vi "flow meter test.vi"() -> ()   [LabVIEW 2013]
uses:
  <vilib>/Platform/TimedLoop/XDataNode/timing_clust.ctl
  <vilib>/Platform/TimedLoop/XDataNode/nitl_modes.ctl
  <vilib>/Platform/TimedLoop/XDataNode/wakeup.ctl
  <vilib>/rvi/Emulation/niFpgaSctlEmulationGetInTimedLoop.vi
  <vilib>/rvi/Emulation/niFpgaEmulationReportErrorSimple.vi
  <vilib>/rvi/Emulation/niFpgaGetClockAttributes.vi
  <vilib>/rvi/Emulation/niFpgaCriticalErrorInLSC.vi
  <vilib>/rvi/eio/common/nirviEmuTemplateMethod_errors.vi
  <vilib>/Platform/TimedLoop/XDataNode/XDataNode.xnode
  <vilib>/eio/EIONode/EIONode.xnode
  <vilib>/Platform/TimedLoop/XDataNode/XDNodeRunTimeDep.lvlib
panel:
  out "Period 6 (ticks)":u32
  out "Period 5 (ticks)":u32
  out "Period 4 (ticks)":u32
  out "Period 3 (ticks)":u32
  out "Period 2 (ticks)":u32
  in  "Max Period (ticks)":u32
  out "Period 1 (ticks)":u32
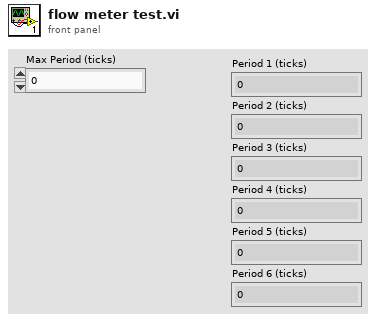
[diagram p1: front panel]
types:
  T1 = typedef "XDNodeRunTimeDep.lvlib/timing_clust.ctl" = cluster{"Expected End [f-1]":u64, "Actual End [f-1]":u64, "Finished Late? [f-1]":bool, "Expected End [i-1]":u64, "Actual End [i-1]":u64, "Finished Late? [i-1]":bool, "Expected Start [i]":u64, "Actual Start [i]":u64, "Expected Start [f]":u64, "Actual Start [f]":u64, "Source Name":string, "Structure Name":string, "Period":i64, "Deadline":i64, "Offset":i64, "Start":i64, "Priority":i32, "Timeout":i32, "Mode":T2, "Wakeup Reason":T3, "Error":errorcluster, "Source Type":string, "Secondary Source Type":string, "Global End Time":u64, "Global Start Time":u64, "Frame Duration":u64, "Iteration Duration":u64, "Assigned CPU":i32, "I/O Scan Engine Mode":u32}
  T2 = typedef "XDNodeRunTimeDep.lvlib/nitl_modes.ctl" = enum32{"No Change", "Process missed periods, maintain original phase", "Discard missed periods, maintain original phase", "Process missed periods, ignore original phase", "Discard missed periods, ignore original phase"}
  T3 = typedef "XDNodeRunTimeDep.lvlib/wakeup.ctl" = enum32{"Normal", "Aborted", "Asynchronous wakeup", "Timing source error", "Timed loop error", "Timeout"}
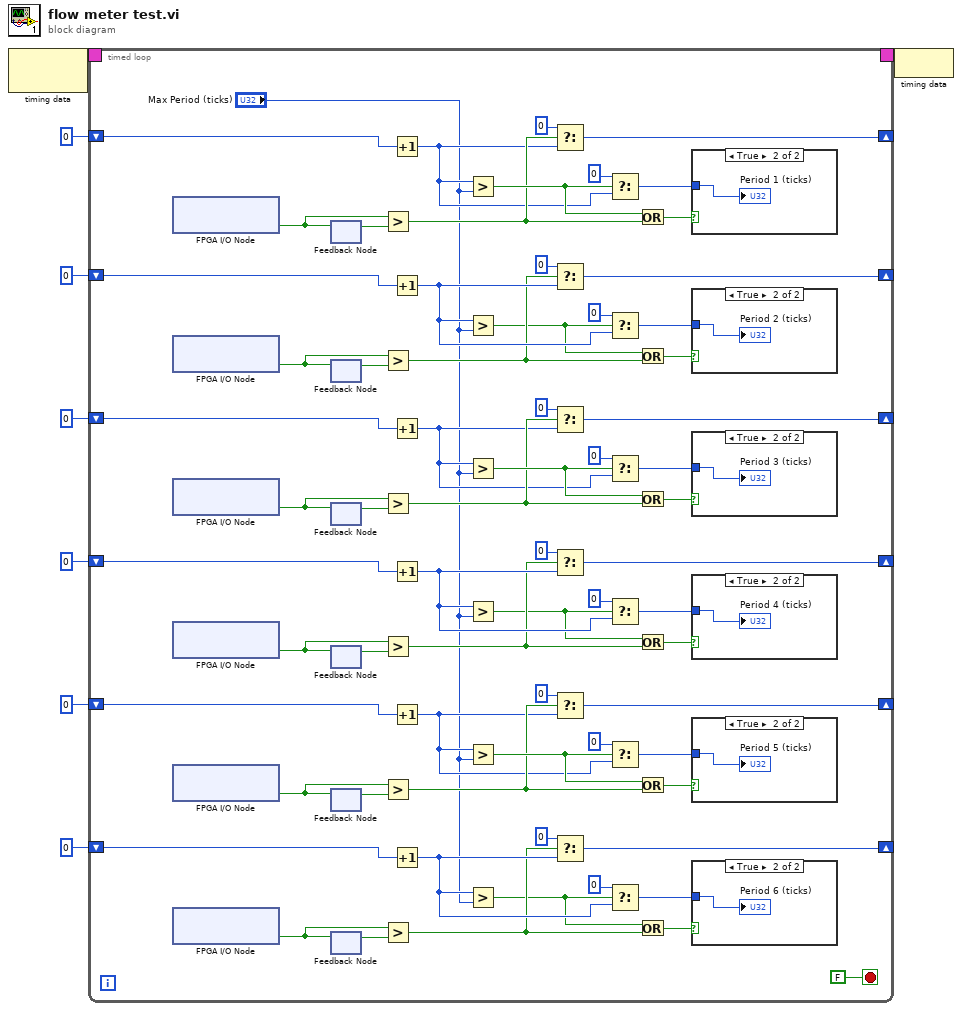
[diagram p0: block diagram]
diagram:
  n1 = node-c288() -> (w8:T1)  [unwired: 1 in]
  n2 = timed-loop {
    timing: w8 -> [_]
    timing-out: [_] -> w7
    shift-right: [w67] -> _
    shift-left: u32 0 ("f") -> [w66]
    shift-right: [w62] -> _
    shift-left: u32 0 ("f") -> [w63]
    shift-right: [w45] -> _
    shift-left: u32 0 ("f") -> [w44]
    shift-right: [w40] -> _
    shift-left: u32 0 ("f") -> [w41]
    shift-right: [w23] -> _
    shift-left: u32 0 ("f") -> [w22]
    shift-right: [w18] -> _
    shift-left: u32 0 ("f") -> [w19]
    stop <- FALSE stop-if-true
    n3 = xnode "FPGA I/O Node"() -> ("RMC/DIO32"=w75:bool)  [unwired: 1 in, 1 out]
    n4 = xnode "FPGA I/O Node"() -> ("RMC/DIO33"=w54:bool)  [unwired: 1 in, 1 out]
    n5 = xnode "FPGA I/O Node"() -> ("RMC/DIO34"=w53:bool)  [unwired: 1 in, 1 out]
    n6 = xnode "FPGA I/O Node"() -> ("RMC/DIO35"=w32:bool)  [unwired: 1 in, 1 out]
    n7 = xnode "FPGA I/O Node"() -> ("RMC/DIO36"=w31:bool)  [unwired: 1 in, 1 out]
    n8 = xnode "FPGA I/O Node"() -> ("RMC/DIO37"=w10:bool)  [unwired: 1 in, 1 out]
    n9 = feedback-in #1(w75) -> ()
    n10 = feedback #1() -> (w74:bool)  [unwired: 1 in]
    n11 = feedback #2() -> (w55:bool)  [unwired: 1 in]
    n12 = feedback-in #2(w54) -> ()
    n13 = feedback #3() -> (w52:bool)  [unwired: 1 in]
    n14 = feedback-in #3(w53) -> ()
    n15 = feedback #4() -> (w33:bool)  [unwired: 1 in]
    n16 = feedback-in #4(w32) -> ()
    n17 = feedback #5() -> (w30:bool)  [unwired: 1 in]
    n18 = feedback-in #5(w31) -> ()
    n19 = feedback #6() -> (w11:bool)  [unwired: 1 in]
    n20 = feedback-in #6(w10) -> ()
    n21 = Greater?(x=w75, y=w74) -> (0:w69:bool)
    n22 = Greater?(x=w54, y=w55) -> (0:w60:bool)
    n23 = Greater?(x=w53, y=w52) -> (0:w47:bool)
    n24 = Greater?(x=w32, y=w33) -> (0:w38:bool)
    n25 = Greater?(x=w31, y=w30) -> (0:w25:bool)
    n26 = Greater?(x=w10, y=w11) -> (0:w16:bool)
    n27 = Increment(x=w66) -> (x+1=w65:u32)
    n28 = Increment(x=w63) -> (x+1=w64:u32)
    n29 = Increment(x=w44) -> (x+1=w43:u32)
    n30 = Increment(x=w41) -> (x+1=w42:u32)
    n31 = Increment(x=w22) -> (x+1=w21:u32)
    n32 = Increment(x=w19) -> (x+1=w20:u32)
    n33 = Greater?(x=w65, y="Max Period (ticks)") -> (0:w71:bool)
    n34 = Greater?(x=w64, y="Max Period (ticks)") -> (0:w58:bool)
    n35 = Greater?(x=w43, y="Max Period (ticks)") -> (0:w49:bool)
    n36 = Greater?(x=w42, y="Max Period (ticks)") -> (0:w36:bool)
    n37 = Greater?(x=w21, y="Max Period (ticks)") -> (0:w27:bool)
    n38 = Greater?(x=w20, y="Max Period (ticks)") -> (0:w14:bool)
    n39 = Select(t=u32 0 ("f"), s=w69, f=w65) -> (s? t:f=w67:u32)
    n40 = Select(t=u32 0 ("f"), s=w60, f=w64) -> (s? t:f=w62:u32)
    n41 = Select(t=u32 0 ("f"), s=w47, f=w43) -> (s? t:f=w45:u32)
    n42 = Select(t=u32 0 ("f"), s=w38, f=w42) -> (s? t:f=w40:u32)
    n43 = Select(t=u32 0 ("f"), s=w25, f=w21) -> (s? t:f=w23:u32)
    n44 = Select(t=u32 0 ("f"), s=w16, f=w20) -> (s? t:f=w18:u32)
    n45 = Select(t=u32 0 ("f"), s=w71, f=w65) -> (s? t:f=w73:u32)
    n46 = Select(t=u32 0 ("f"), s=w58, f=w64) -> (s? t:f=w56:u32)
    n47 = Select(t=u32 0 ("f"), s=w49, f=w43) -> (s? t:f=w51:u32)
    n48 = Select(t=u32 0 ("f"), s=w36, f=w42) -> (s? t:f=w34:u32)
    n49 = Select(t=u32 0 ("f"), s=w27, f=w21) -> (s? t:f=w29:u32)
    n50 = Select(t=u32 0 ("f"), s=w14, f=w20) -> (s? t:f=w12:u32)
    n51 = Or(x=w71, y=w69) -> (x .or. y?=w70:bool)
    n52 = Or(x=w58, y=w60) -> (x .or. y?=w59:bool)
    n53 = Or(x=w49, y=w47) -> (x .or. y?=w48:bool)
    n54 = Or(x=w36, y=w38) -> (x .or. y?=w37:bool)
    n55 = Or(x=w27, y=w25) -> (x .or. y?=w26:bool)
    n56 = Or(x=w14, y=w16) -> (x .or. y?=w15:bool)
    n57 = case shown="True" w70 {
      tunnel: w73 -> [_ w82]
      frame False {
      }
      frame True {
        "Period 1 (ticks)" <- w82
      }
    }
    n58 = case shown="True" w59 {
      tunnel: w56 -> [_ w81]
      frame False {
      }
      frame True {
        "Period 2 (ticks)" <- w81
      }
    }
    n59 = case shown="True" w48 {
      tunnel: w51 -> [_ w80]
      frame False {
      }
      frame True {
        "Period 3 (ticks)" <- w80
      }
    }
    n60 = case shown="True" w37 {
      tunnel: w34 -> [_ w79]
      frame False {
      }
      frame True {
        "Period 4 (ticks)" <- w79
      }
    }
    n61 = case shown="True" w26 {
      tunnel: w29 -> [_ w78]
      frame False {
      }
      frame True {
        "Period 5 (ticks)" <- w78
      }
    }
    n62 = case shown="True" w15 {
      tunnel: w12 -> [_ w77]
      frame False {
      }
      frame True {
        "Period 6 (ticks)" <- w77
      }
    }
  }
  n63 = node-c288(w7) -> ()
